vi "Save as FITS.vi"(8 "error in (no error)":errorcluster, 11 "CCDCamera in":refnum<class "CCDCamera.lvclass">) -> (0 "error out":errorcluster, 3 "CCDCamera out":refnum<class "CCDCamera.lvclass">)   [LabVIEW 2018, in "CCDCamera.lvclass"]
uses:
  CCDCamera.lvclass
  <userlib>/atmcd32d.llb/FITS_type typedef.ctl
  CCDCamera.lvclass/CCDCamera.ctl
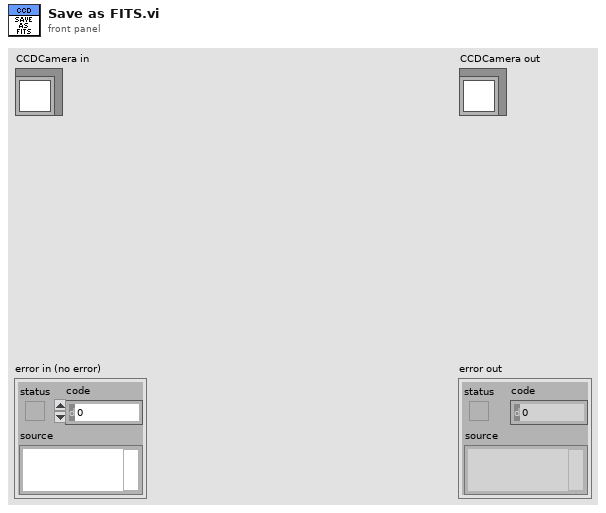
[diagram p1: front panel]
types:
  T1 = typedef "FITS_type typedef.ctl" = enum16{"Unsigned 16", "Unsigned 32", "Signed 16", "Signed 32", "Float"}
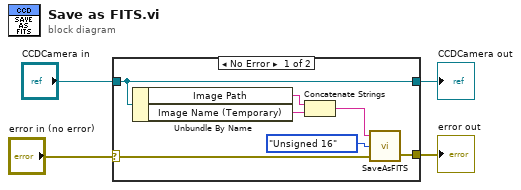
[diagram p0: block diagram]
diagram:
  n1 = case shown="No Error" "error in (no error)" {
    selector: "error in (no error)" -> [w10 w13]
    tunnel: [w9 w13] -> w3
    tunnel: [w8 w12] -> w1
    tunnel: "CCDCamera in" -> [w8 w12]
    frame No Error {
      n2 = Unbundle By Name(w8) -> ("Image Path"=w7:string, "Image Name (Temporary)"=w6:string)
      n3 = Concatenate Strings(w7, w6) -> (w5:string)
      n4 = call <userlib>:"SaveAsFITS.vi"("error in (no error)"=w10, "FITS_type"=FITS_type_typedef."Unsigned 16", "path"=w5) -> ("error out"=w9:errorcluster)  [unwired: 1 out]
    }
    frame Error {
    }
  }
  "error out" <- w3
  "CCDCamera out" <- w1
